vi "SubConfocal_SetShutterStatus.vi"(7 "Confocal scanner":T1={"SDC shutter"=FALSE, "Filter wheel"=3, "FW speed"=3, "Disk spinning"=FALSE, "Disk speed (rpm)"=3000.0} {"Disk speed (rpm)" min=1500.0 max=10000.0; "FW speed" min=1 max=5 step=1; "Filter wheel" items=["CFP"=1, "GFP"=2, "mCherry"=3, "Alexa-647"=4, "OFP"=5, "empty"=6]}, 8 "Error In":errorcluster, 11 "Confocal line (VISA IN)":refnum<visa-resource-name>="COM1") -> (0 "Error out":errorcluster, 3 "VISA OUT":refnum<visa-resource-name>="COM1")   [LabVIEW 2015]
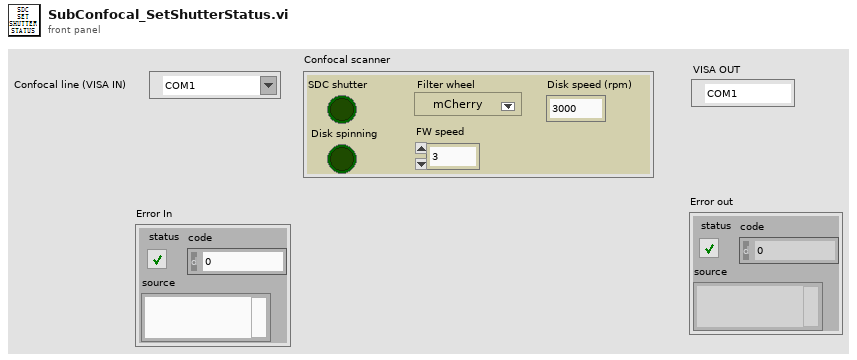
[diagram p1: front panel]
types:
  T1 = cluster{"SDC shutter":bool, "Filter wheel":u16, "FW speed":i32, "Disk spinning":bool, "Disk speed (rpm)":dbl}
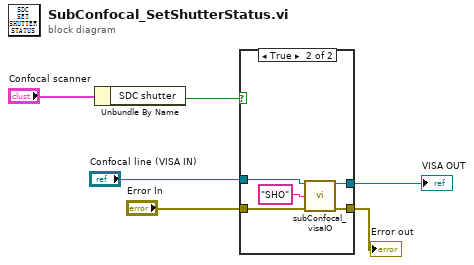
[diagram p0: block diagram]
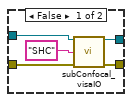
[diagram p2: hidden frame]
diagram:
  n1 = Unbundle By Name("Confocal scanner") -> ("SDC shutter"=w1:bool)
  n2 = case shown="True" w1 {
    tunnel: [w9 w16] -> w5
    tunnel: "Confocal line (VISA IN)" -> [w10 w14]
    tunnel: "Error In" -> [w8 w13]
    tunnel: [w7 w12] -> w3
    frame False {
      n3 = call "subConfocal_visaIO.vi"("VISA  IN"=w10, "Command (to ctlr)"="SHC", "error in"=w8) -> ("VISA OUT"=w9:refnum<visa-resource-name>, "error out"=w7:errorcluster)  [unwired: 8 in, 3 out]
    }
    frame True {
      n4 = call "subConfocal_visaIO.vi"("VISA  IN"=w14, "Command (to ctlr)"="SHO", "error in"=w13) -> ("VISA OUT"=w16:refnum<visa-resource-name>, "error out"=w12:errorcluster)  [unwired: 8 in, 3 out]
    }
  }
  "VISA OUT" <- w5
  "Error out" <- w3
